vi "handler_laser.vi"(8 "error in (no error)":errorcluster, 11 "HTTP Request in":T1) -> (0 "error out":errorcluster, 1 "Handler name":string, 3 "HTTP Request out":T1)   [LabVIEW 2011]
uses:
  http_field.ctl
  http_request.ctl
  http_response.ctl
  template_field_type.ctl
  template_field.ctl
  http_request_response.ctl
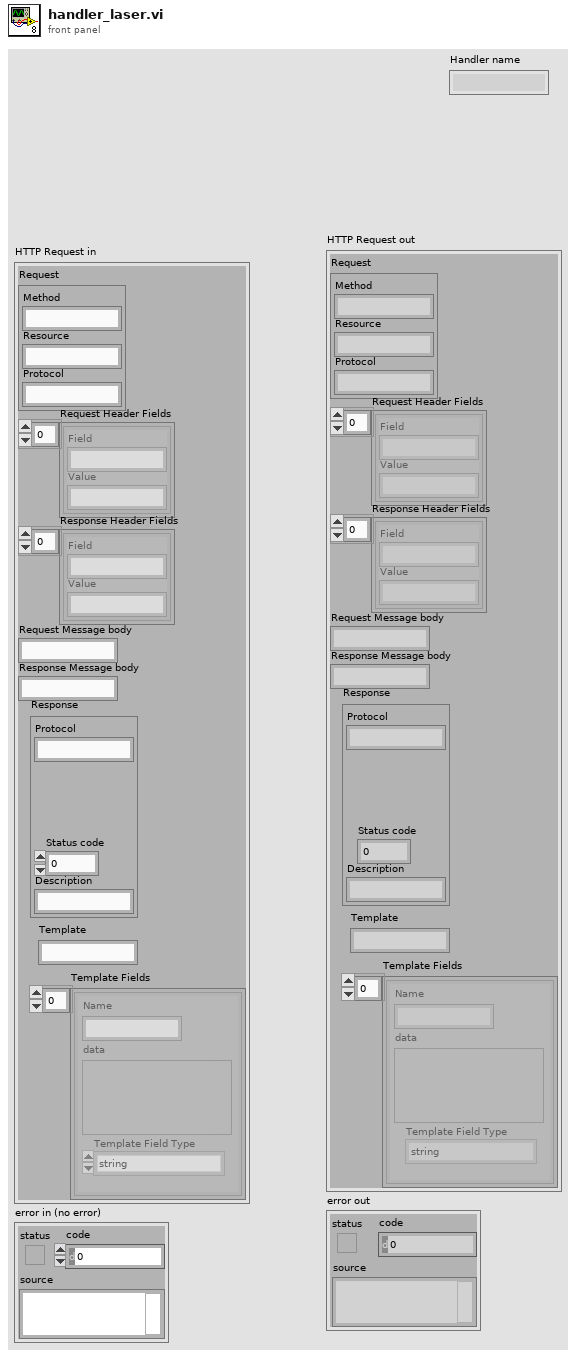
[diagram p1: front panel]
types:
  T1 = typedef "http_request_response.ctl" = cluster{"Request":T2, "Request Header Fields":T3[], "Response Header Fields":T3[], "Request Message body":string, "Response Message body":string, "Response":T4, "Template":string, "Template Fields":T5[]}
  T2 = typedef "http_request.ctl" = cluster{"Method":string, "Resource":string, "Protocol":string}
  T3 = typedef "http_field.ctl" = cluster{"Field":string, "Value":string}
  T4 = typedef "http_response.ctl" = cluster{"Protocol":string, "Status code":dbl, "Description":string}
  T5 = typedef "template_field.ctl" = cluster{"Name":string, "Template Field Type":T6, "data":variant}
  T6 = typedef "template_field_type.ctl" = enum16{"string", "string array", "number", "number array", "cluster", "cluster array"}
  T7 = typedef "html_form_field.ctl" = cluster{"field name":string, "field value":string}
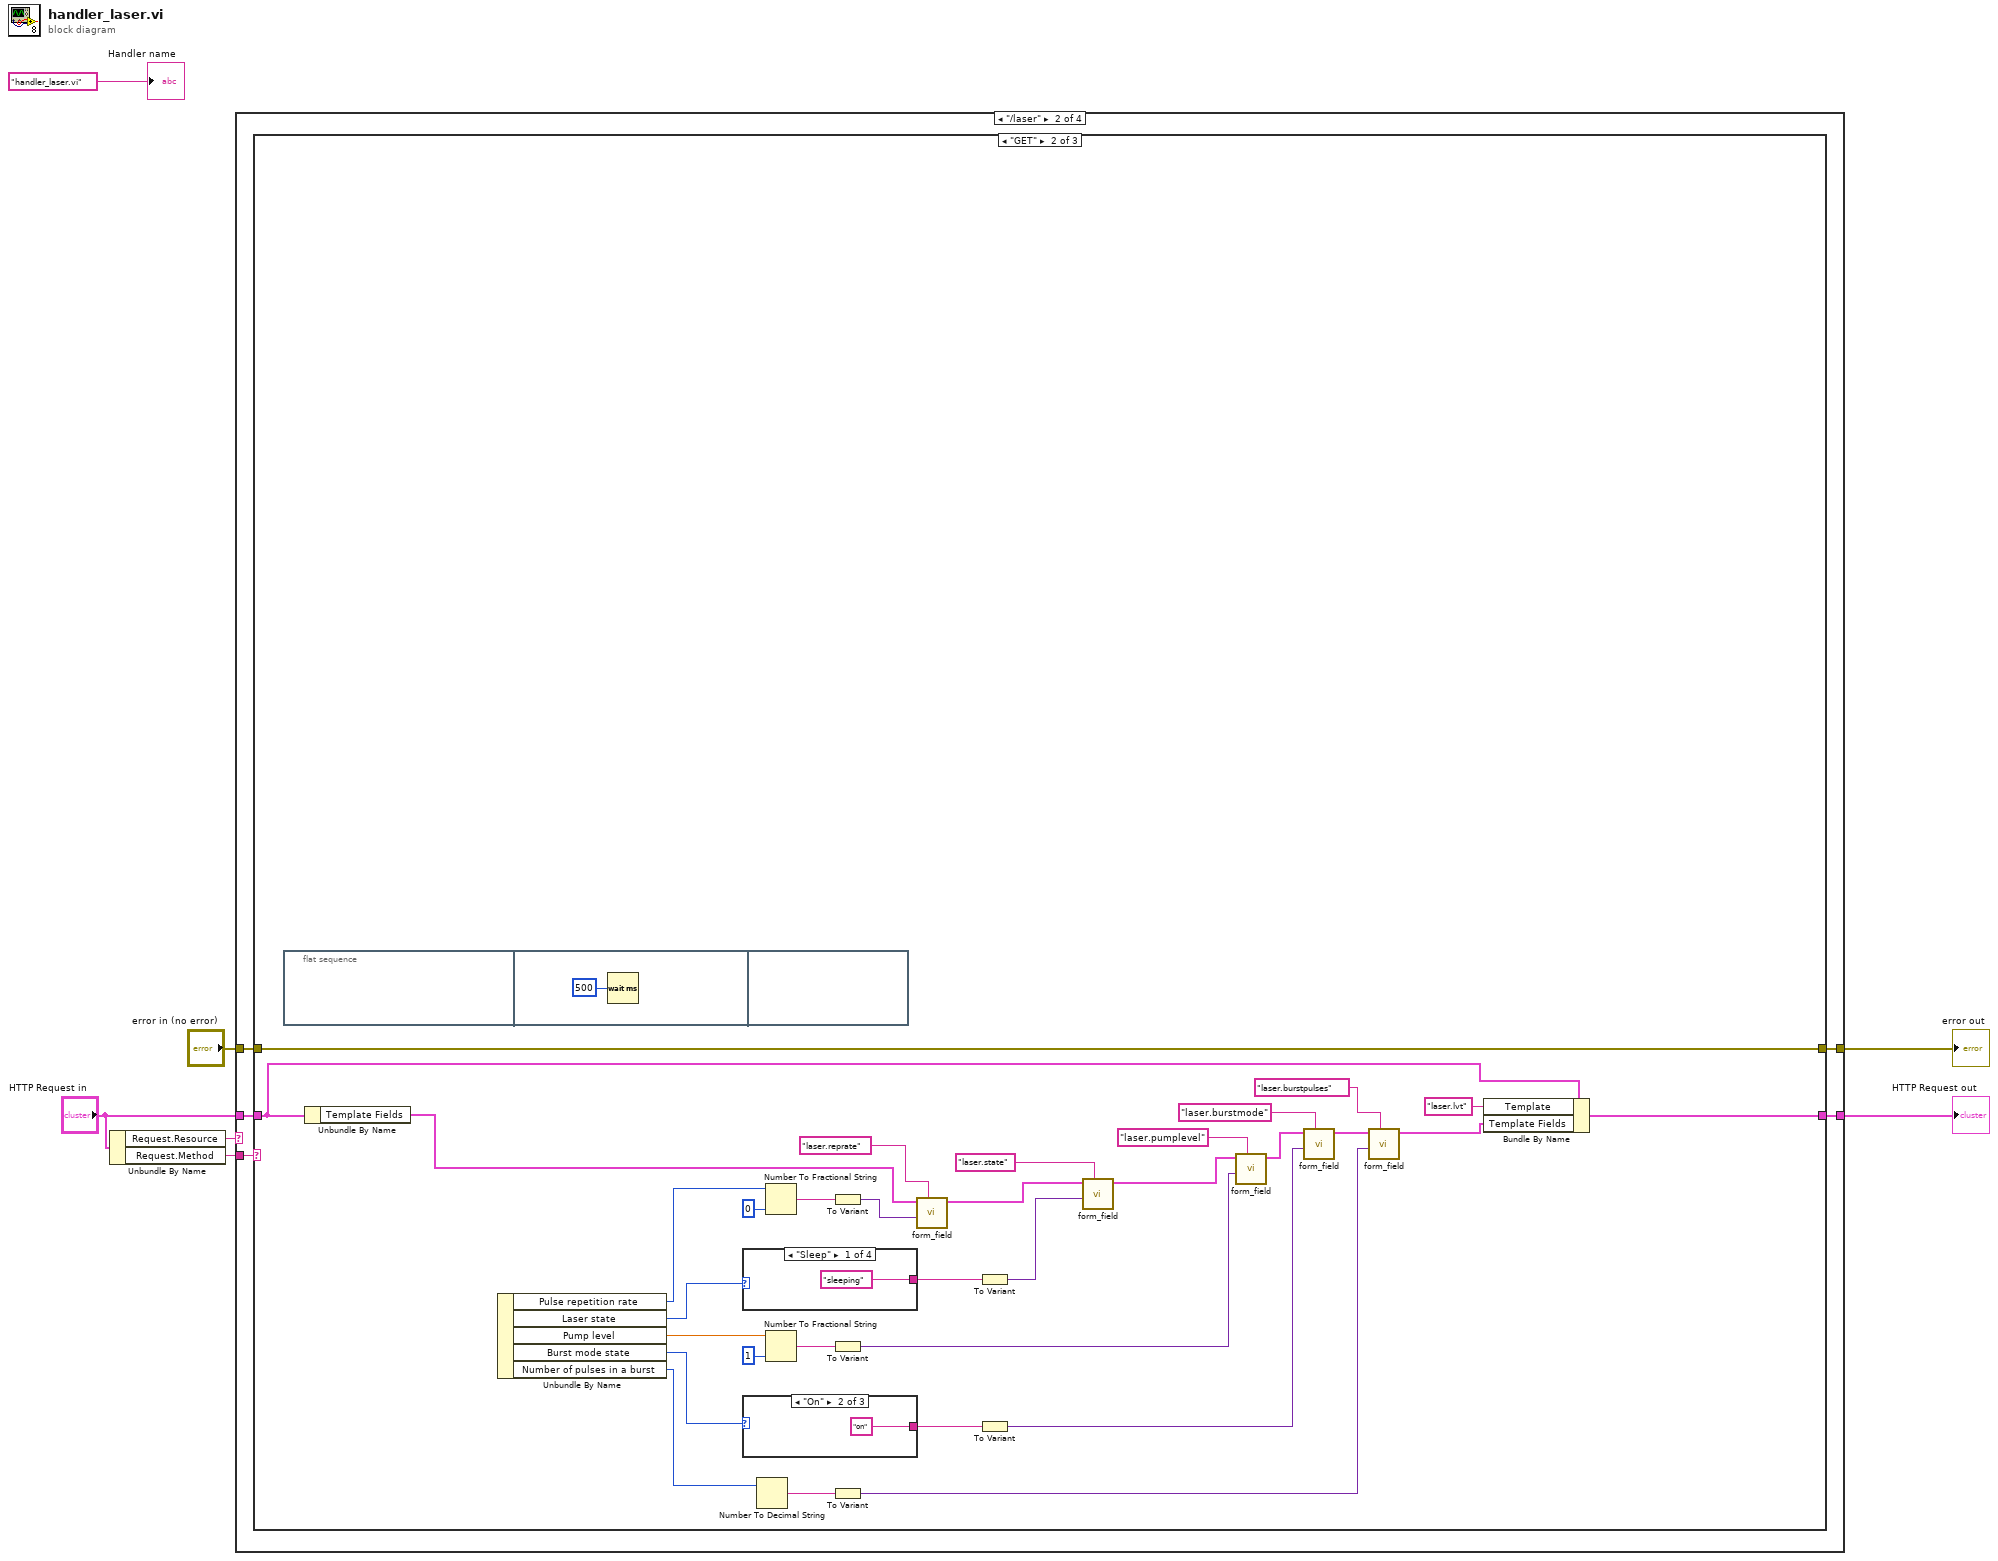
[diagram p0: block diagram]
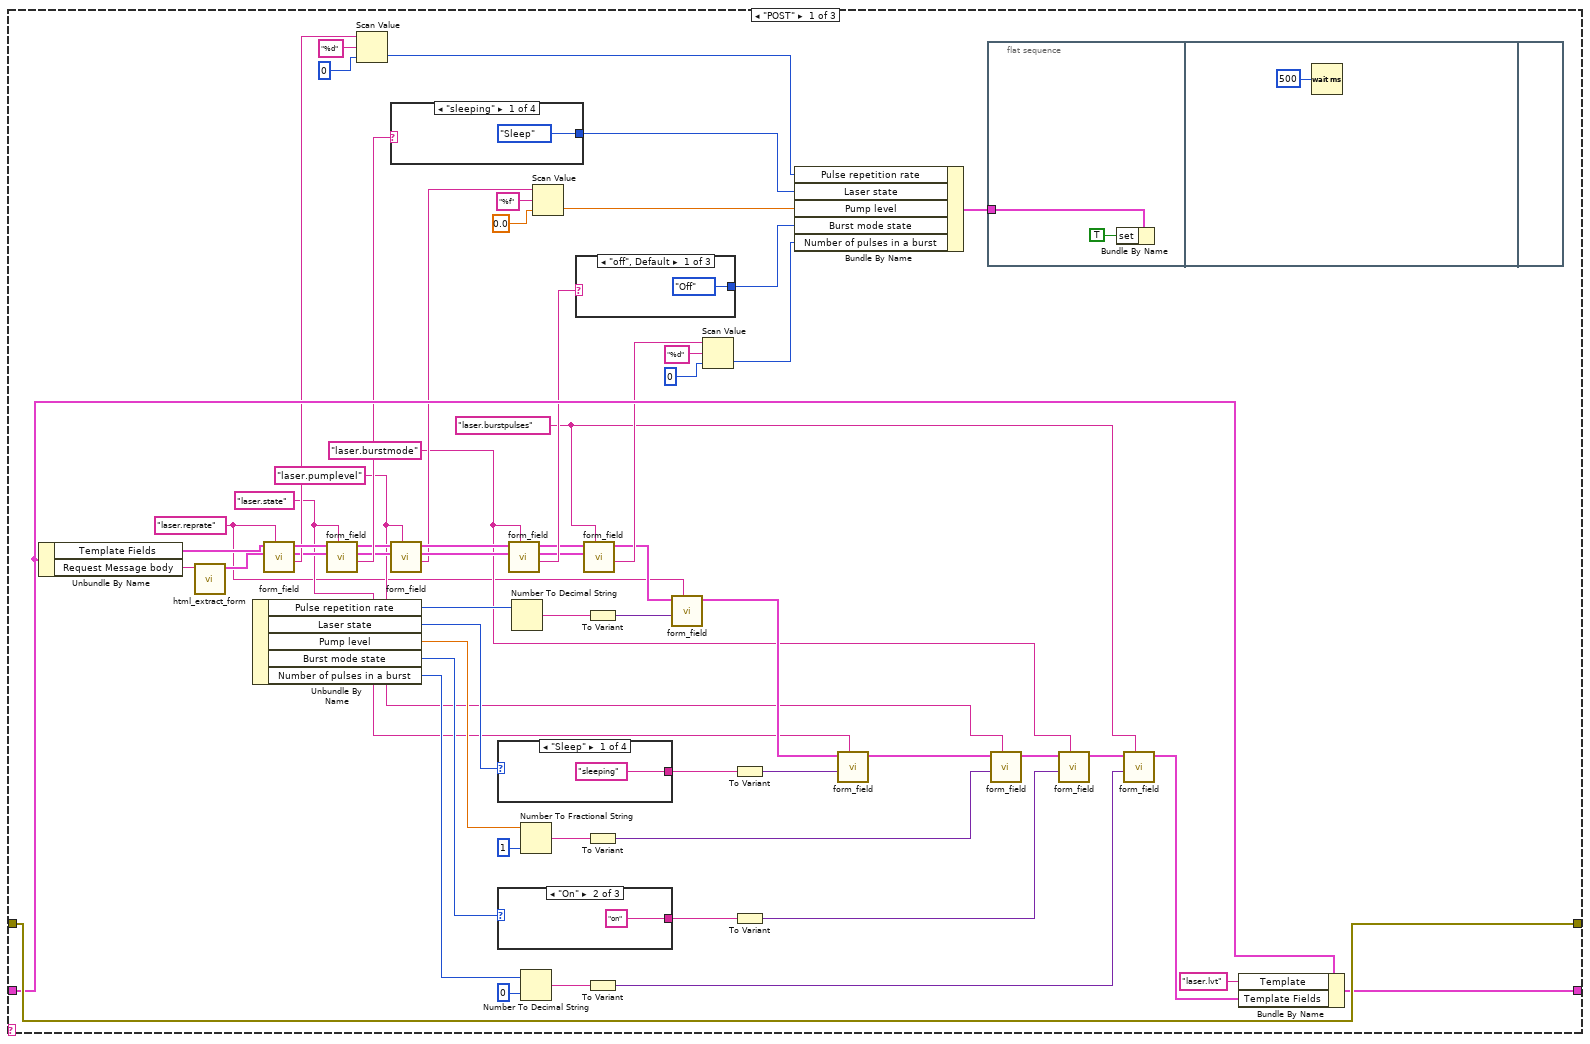
[diagram p3: hidden frame]
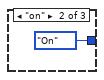
[diagram p4: hidden frame]
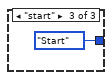
[diagram p5: hidden frame]
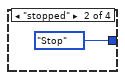
[diagram p6: hidden frame]
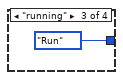
[diagram p7: hidden frame]
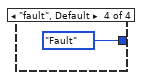
[diagram p8: hidden frame]
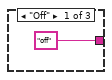
[diagram p9: hidden frame]
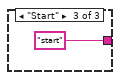
[diagram p10: hidden frame]
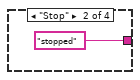
[diagram p11: hidden frame]
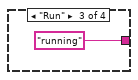
[diagram p12: hidden frame]
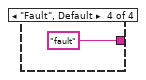
[diagram p13: hidden frame]
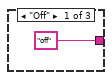
[diagram p14: hidden frame]
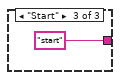
[diagram p15: hidden frame]
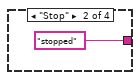
[diagram p16: hidden frame]
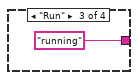
[diagram p17: hidden frame]
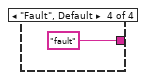
[diagram p18: hidden frame]
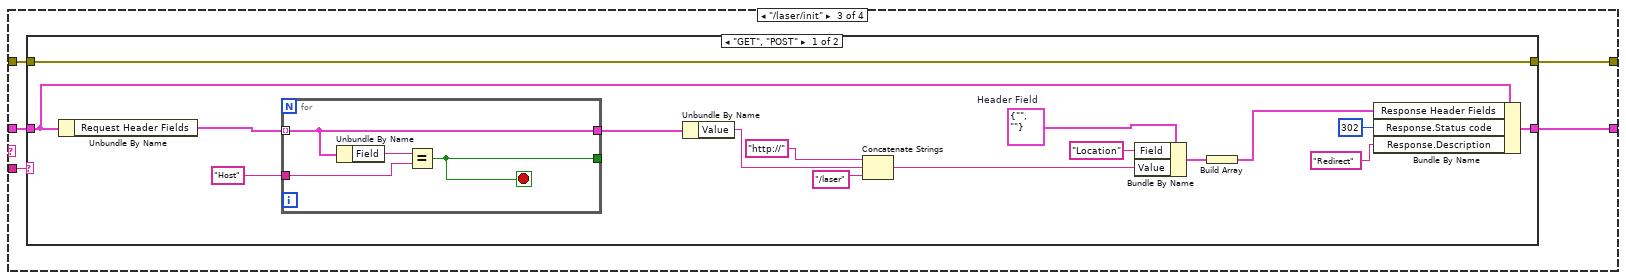
[diagram p20: hidden frame]
diagram:
  n1 = Unbundle By Name("HTTP Request in") -> ("Request.Resource"=w7:string, "Request.Method"=w6:string)
  n2 = case shown="\"/laser\"" w7 {
    tunnel: w6 -> [_ w14 w138 w165]
    tunnel: "HTTP Request in" -> [w9 w13 w137 w164]
    tunnel: [w9 w12 w136 w163] -> w3
    tunnel: "error in (no error)" -> [w8 w11 w135 w162]
    tunnel: [w8 w10 w134 w161] -> w2
    frame Default {
    }
    frame "/laser" {
      n3 = case shown="\"GET\"" w14 {
        tunnel: w13 -> [w60 w120 w133]
        tunnel: [w59 w122 w133] -> w12
        tunnel: w11 -> [w74 w123 w132]
        tunnel: [w74 w123 w132] -> w10
        frame "POST" {
          w19 = "laser.burstpulses" ("Name")
          w18 = "laser.burstmode" ("Name")
          w17 = "laser.pumplevel" ("Name")
          w16 = "laser.state" ("Name")
          w15 = "laser.reprate" ("Name")
          n4 = Unbundle By Name(w60) -> ("Template Fields"=w45:T5[], "Request Message body"=w58:string)
          n5 = call "html_extract_form.vi"("Message Body"=w58) -> ("Form Data"=w44:T7[])  [unwired: 10 in]
          n6 = Unbundle By Name() -> ("Pulse repetition rate"=w70:u16, "Laser state"=w69:enum16{"Sleep", "Stop", "Run", "Fault"}, "Pump level"=w62:dbl, "Burst mode state"=w67:enum16{"Off", "On", "Start"}, "Number of pulses in a burst"=w66:u32)  [unwired: 1 in]
          n7 = call "form_field.vi"("Name"=w15, "Form Data"=w44, "Template Fields"=w45) -> ("field value"=w42:string, "Form Data"=w41:T7[], "Template Fields"=w43:T5[])  [unwired: 6 in]
          n8 = call "form_field.vi"("Name"=w16, "Form Data"=w41, "Template Fields"=w43) -> ("field value"=w40:string, "Form Data"=w38:T7[], "Template Fields"=w39:T5[])  [unwired: 6 in]
          n9 = Scan Value(string=w42, format string="%d", default (0 dbl)=u16 0) -> (value=w56:u16)  [unwired: 1 out]
          n10 = case shown="\"sleeping\"" w40 {
            tunnel: [enum16{"Sleep", "Stop", "Run", "Fault"}."Sleep" ("Laser state") enum16{"Sleep", "Stop", "Run", "Fault"}."Stop" ("Laser state") enum16{"Sleep", "Stop", "Run", "Fault"}."Run" ("Laser state") enum16{"Sleep", "Stop", "Run", "Fault"}."Fault" ("Laser state")] -> w47
            frame "sleeping" {
            }
            frame "stopped" {
            }
            frame "running" {
            }
            frame "fault", Default {
            }
          }
          n11 = call "form_field.vi"("Name"=w17, "Form Data"=w38, "Template Fields"=w39) -> ("field value"=w35:string, "Form Data"=w36:T7[], "Template Fields"=w37:T5[])  [unwired: 6 in]
          n12 = case shown="\"Sleep\"" w69 {
            tunnel: ["sleeping" "stopped" "running" "fault"] -> w68
            frame "Sleep" {
            }
            frame "Stop" {
            }
            frame "Run" {
            }
            frame "Fault", Default {
            }
          }
          n13 = case shown="\"On\"" w67 {
            tunnel: ["off" "on" "start"] -> w64
            frame "Off" {
            }
            frame "On" {
            }
            frame "Start" {
            }
          }
          n14 = call "form_field.vi"("Name"=w18, "Form Data"=w36, "Template Fields"=w37) -> ("field value"=w34:string, "Form Data"=w32:T7[], "Template Fields"=w33:T5[])  [unwired: 6 in]
          n15 = Number To Decimal String(number=w70) -> (decimal integer string=w72:string)  [unwired: 1 in]
          n16 = Number To Fractional String(number=w62, precision (6)=i16 1) -> (F-format string=w63:string)  [unwired: 2 in]
          n17 = Number To Decimal String(number=w66, width (-)=i16 0 ("precision (6)")) -> (decimal integer string=w71:string)
          n18 = Scan Value(string=w35, format string="%f", default (0 dbl)=0.0) -> (value=w52:dbl)  [unwired: 1 out]
          n19 = case shown="\"off\", Default" w34 {
            tunnel: [enum16{"Off", "On", "Start"}."Off" ("Burst mode state") enum16{"Off", "On", "Start"}."On" ("Burst mode state") enum16{"Off", "On", "Start"}."Start" ("Burst mode state")] -> w48
            frame "off", Default {
            }
            frame "on" {
            }
            frame "start" {
            }
          }
          n20 = call "form_field.vi"("Name"=w19, "Form Data"=w32, "Template Fields"=w33) -> ("field value"=w31:string, "Template Fields"=w30:T5[])  [unwired: 6 in, 1 out]
          n21 = To Variant(anything=w72) -> (Variant=w24:variant)
          n22 = To Variant(anything=w63) -> (Variant=w22:variant)
          n23 = To Variant(anything=w71) -> (Variant=w20:variant)
          n24 = call "form_field.vi"("Name"=w15, "Value"=w24, "Template Fields"=w30) -> ("Template Fields"=w29:T5[])  [unwired: 6 in, 2 out]
          n25 = Scan Value(string=w31, format string="%d", default (0 dbl)=u16 0) -> (value=w49:u16)  [unwired: 1 out]
          n26 = To Variant(anything=w68) -> (Variant=w23:variant)
          n27 = To Variant(anything=w64) -> (Variant=w21:variant)
          n28 = Bundle By Name("Pulse repetition rate"=w56, "Laser state"=w47, "Pump level"=w52, "Burst mode state"=w48, "Number of pulses in a burst"=w49) -> (w46:cluster{})  [unwired: 1 in]
          n29 = call "form_field.vi"("Name"=w16, "Value"=w23, "Template Fields"=w29) -> ("Template Fields"=w28:T5[])  [unwired: 6 in, 2 out]
          n30 = flat-sequence {
            tunnel: w46 -> [w75]
            frame #0 {
              n31 = Bundle By Name(cluster=w75, "set"=TRUE ("get")) -> ()  [unwired: 1 out]
            }
            frame #1 {
              n32 = Wait (ms)(milliseconds to wait=u32 500) -> ()  [unwired: 1 out]
            }
            frame #2 {
            }
          }
          n33 = call "form_field.vi"("Name"=w17, "Value"=w22, "Template Fields"=w28) -> ("Template Fields"=w27:T5[])  [unwired: 6 in, 2 out]
          n34 = call "form_field.vi"("Name"=w18, "Value"=w21, "Template Fields"=w27) -> ("Template Fields"=w26:T5[])  [unwired: 6 in, 2 out]
          n35 = call "form_field.vi"("Name"=w19, "Value"=w20, "Template Fields"=w26) -> ("Template Fields"=w25:T5[])  [unwired: 6 in, 2 out]
          n36 = Bundle By Name(cluster=w60, "Template"="laser.lvt", "Template Fields"=w25) -> (w59:T1)
        }
        frame "GET" {
          n37 = flat-sequence {
            frame #0 {
            }
            frame #1 {
              n38 = Wait (ms)(milliseconds to wait=u32 500) -> ()  [unwired: 1 out]
            }
            frame #2 {
            }
          }
          n39 = Unbundle By Name(w120) -> ("Template Fields"=w107:T5[])
          n40 = Unbundle By Name() -> ("Pulse repetition rate"=w117:u16, "Laser state"=w115:enum16{"Sleep", "Stop", "Run", "Fault"}, "Pump level"=w109:dbl, "Burst mode state"=w113:enum16{"Off", "On", "Start"}, "Number of pulses in a burst"=w112:u32)  [unwired: 1 in]
          n41 = case shown="\"Sleep\"" w115 {
            tunnel: ["sleeping" "stopped" "running" "fault"] -> w114
            frame "Sleep" {
            }
            frame "Stop" {
            }
            frame "Run" {
            }
            frame "Fault", Default {
            }
          }
          n42 = case shown="\"On\"" w113 {
            tunnel: ["off" "on" "start"] -> w111
            frame "Off" {
            }
            frame "On" {
            }
            frame "Start" {
            }
          }
          n43 = Number To Decimal String(number=w112) -> (decimal integer string=w118:string)  [unwired: 1 in]
          n44 = Number To Fractional String(number=w117, precision (6)=i16 0) -> (F-format string=w119:string)  [unwired: 2 in]
          n45 = Number To Fractional String(number=w109, precision (6)=i16 1) -> (F-format string=w110:string)  [unwired: 2 in]
          n46 = To Variant(anything=w119) -> (Variant=w95:variant)
          n47 = To Variant(anything=w110) -> (Variant=w96:variant)
          n48 = To Variant(anything=w118) -> (Variant=w92:variant)
          n49 = call "form_field.vi"("Name"="laser.reprate", "Value"=w95, "Template Fields"=w107) -> ("Template Fields"=w106:T5[])  [unwired: 6 in, 2 out]
          n50 = To Variant(anything=w114) -> (Variant=w94:variant)
          n51 = To Variant(anything=w111) -> (Variant=w93:variant)
          n52 = call "form_field.vi"("Name"="laser.state", "Value"=w94, "Template Fields"=w106) -> ("Template Fields"=w105:T5[])  [unwired: 6 in, 2 out]
          n53 = call "form_field.vi"("Name"="laser.pumplevel", "Value"=w96, "Template Fields"=w105) -> ("Template Fields"=w104:T5[])  [unwired: 6 in, 2 out]
          n54 = call "form_field.vi"("Name"="laser.burstmode", "Value"=w93, "Template Fields"=w104) -> ("Template Fields"=w103:T5[])  [unwired: 6 in, 2 out]
          n55 = call "form_field.vi"("Name"="laser.burstpulses", "Value"=w92, "Template Fields"=w103) -> ("Template Fields"=w102:T5[])  [unwired: 6 in, 2 out]
          n56 = Bundle By Name(cluster=w120, "Template"="laser.lvt", "Template Fields"=w102) -> (w122:T1)
        }
        frame Default {
        }
      }
    }
    frame "/laser/init" {
      n57 = case shown="\"GET\", \"POST\"" w138 {
        tunnel: w137 -> [w148 w160]
        tunnel: [w153 w160] -> w136
        tunnel: w135 -> [w154 w159]
        tunnel: [w154 w159] -> w134
        frame "GET", "POST" {
          w151 = T3 {"Field"="", "Value"=""}  # Header Field
          n58 = Unbundle By Name(w148) -> ("Request Header Fields"=w147:T3[])
          n59 = for {
            tunnel: w147 -> [w155] mode=indexing
            tunnel: "Host" ("Name") -> [w157]
            tunnel: [w156] -> _
            tunnel: [w155] -> w145
            stop <- w156 stop-if-true
            n60 = Unbundle By Name(w155) -> ("Field"=w158:string)
            n61 = Equal?(x=w158, y=w157) -> (x = y?=w156:bool)
          }
          n62 = Unbundle By Name(w145) -> ("Value"=w144:string)
          n63 = Concatenate Strings("http://" ("string"), w144, "/laser" ("Value")) -> (w142:string)
          n64 = Bundle By Name(cluster=w151, "Field"="Location", "Value"=w142) -> (w150:T3)
          n65 = Build Array(w150) -> (w152:T3[])
          n66 = Bundle By Name(cluster=w148, "Response Header Fields"=w152, "Response.Status code"=u16 302, "Response.Description"="Redirect") -> (w153:T1)
        }
        frame Default {
        }
      }
    }
    frame "/laser/stop" {
      n67 = case shown="\"GET\", \"POST\"" w165 {
        tunnel: w164 -> [w175 w187]
        tunnel: [w180 w187] -> w163
        tunnel: w162 -> [w181 w186]
        tunnel: [w181 w186] -> w161
        frame "GET", "POST" {
          w178 = T3 {"Field"="", "Value"=""}  # Header Field
          n68 = Unbundle By Name(w175) -> ("Request Header Fields"=w174:T3[])
          n69 = for {
            tunnel: w174 -> [w182] mode=indexing
            tunnel: "Host" ("Name") -> [w184]
            tunnel: [w183] -> _
            tunnel: [w182] -> w172
            stop <- w183 stop-if-true
            n70 = Unbundle By Name(w182) -> ("Field"=w185:string)
            n71 = Equal?(x=w185, y=w184) -> (x = y?=w183:bool)
          }
          n72 = Unbundle By Name(w172) -> ("Value"=w171:string)
          n73 = Concatenate Strings("http://" ("string"), w171, "/laser" ("Value")) -> (w169:string)
          n74 = Bundle By Name(cluster=w178, "Field"="Location", "Value"=w169) -> (w177:T3)
          n75 = Build Array(w177) -> (w179:T3[])
          n76 = Bundle By Name(cluster=w175, "Response Header Fields"=w179, "Response.Status code"=u16 302, "Response.Description"="Redirect") -> (w180:T1)
        }
        frame Default {
        }
      }
    }
  }
  "HTTP Request out" <- w3
  "error out" <- w2
  "Handler name" <- "handler_laser.vi" ("Handler name")
